vi "Example Toolbar.vi"() -> ()   [LabVIEW 2011, in "Toolbar Control.lvclass"]
doc: "This is an example VI that demonstrates how to use the Toolbar Control object. Run the VI and following the instructions on the front panel.\n\n-------------\nDeveloped by Brian Hoover (hooovahh)"
uses:
  Toolbar Control.lvclass
  Controls/Button State.ctl
  Controls/Horizontal Initialize Settings.ctl
  Controls/Vertical Initialize Settings.ctl
  <userlib>/_OpenG.lib/file/file.llb/Build Path - File Names Array - path__ogtk.vi
  Public Functions/Add Icons From Paths.vi
  Properties/Read Button Pressed Event.vi
  Properties/Read Draw Toolbar Event.vi
  Properties/Write Picture Control Bounds.vi
  Properties/Write Background Color.vi
panel:
  out "Picture":picture
  in  "Top Pane Color":u32(colorbox)
  out "Icon Index":i32
  out "Button State":T1
  out "Button Pressed":string
  in  "Button State":T1
  in  "Button Index":i32
  in  "Set State":bool
  in  "stop":bool
  # "Run this VI.  A toolbar is made using only PNG images for what the button should look like when the mouse is not over the button.\n\nIf there are too many buttons, a More Options button will be on the right to show the rest in a vertical list.  If the vertical list is too large it will show a scrollbar for the remaining buttons.\n\nButtons can be enabled, disabled, or disabled and greyed out.  And the pane color can be changed and buttons will change to match."
  # "Button Pressed Indicators"
  # "Set Button State Controls"
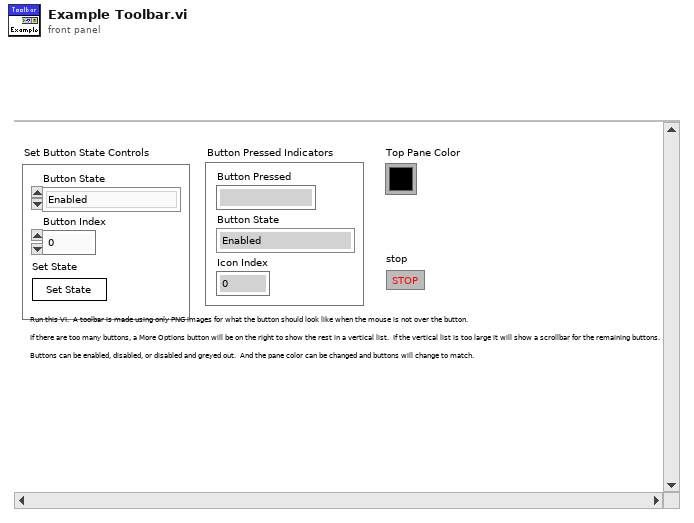
[diagram p1: front panel]
types:
  T1 = typedef "Toolbar Control.lvclass/Button State.ctl" = enum8{"Enabled", "Disabled", "Disabled and Grayed Out"}
  T2 = typedef "Vertical Initialize Settings.ctl" = cluster{"Button Width":i32, "Button Height":i32, "Separator Height":i32}
  T3 = typedef "Horizontal Initialize Settings.ctl" = cluster{"Button Width":i32, "Button Height":i32, "Separator Width":i32, "More Options Width":i32}
  T4 = typedef "LVRectTypeDef.ctl" = cluster{"left":i16, "top":i16, "right":i16, "bottom":i16}
  T5 = typedef "LVPoint32TypeDef.ctl" = cluster{"Horizontal":i32, "Vertical":i32}
  T6 = typedef "Button State.ctl" = enum8{"Enabled", "Disabled", "Disabled and Grayed Out"}
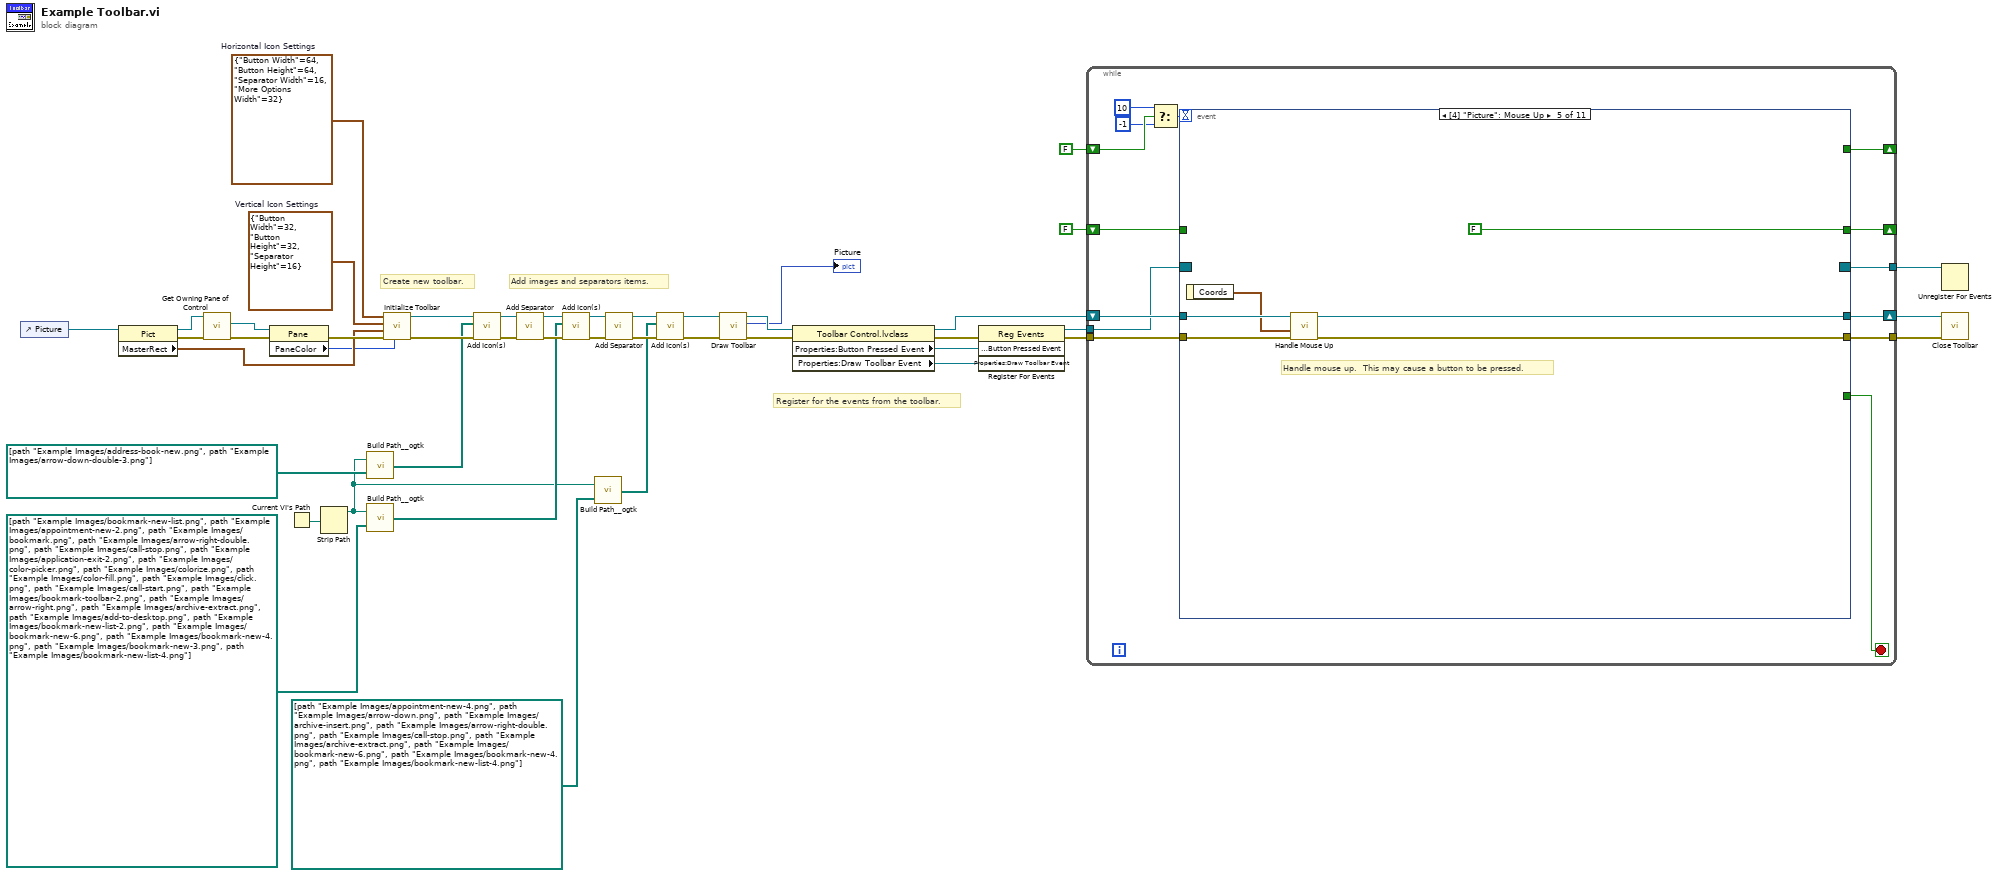
[diagram p0: block diagram]
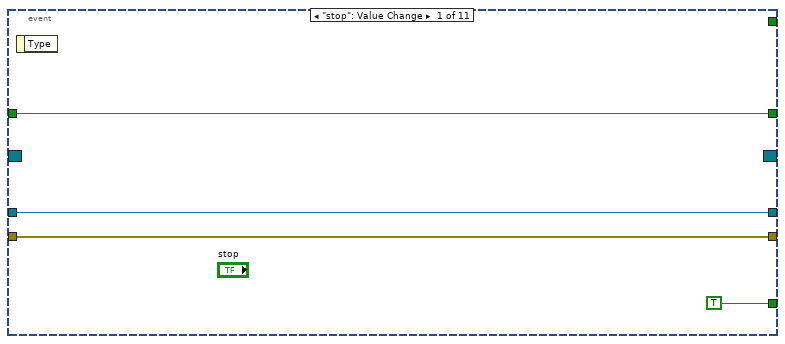
[diagram p2: hidden frame]
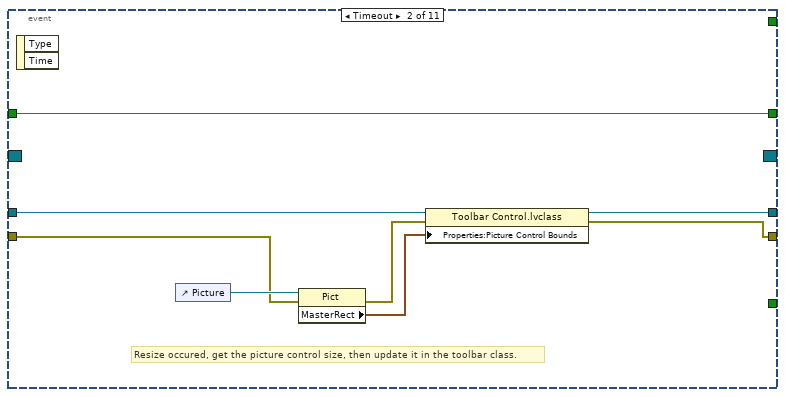
[diagram p3: hidden frame]
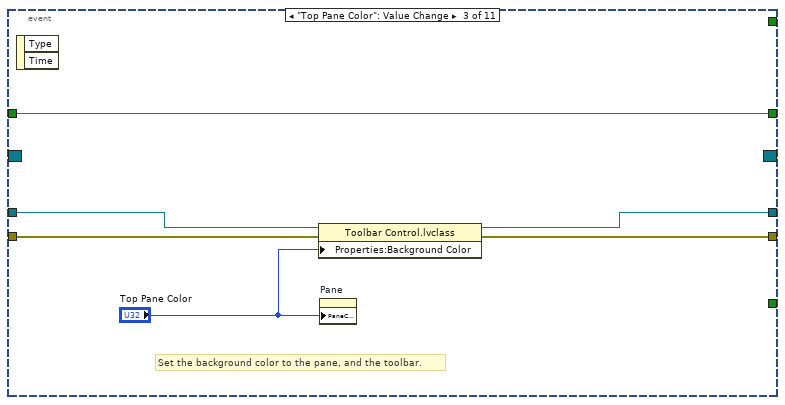
[diagram p4: hidden frame]
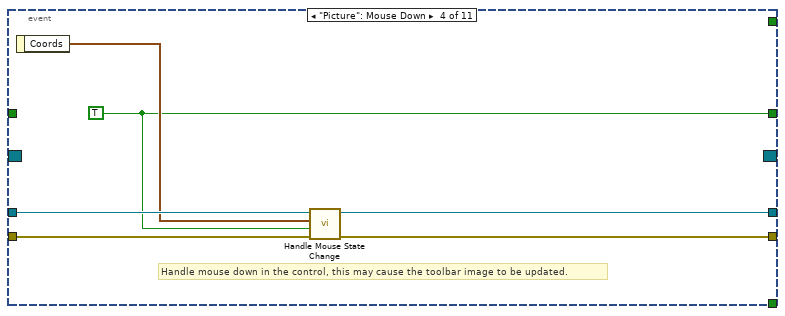
[diagram p5: hidden frame]
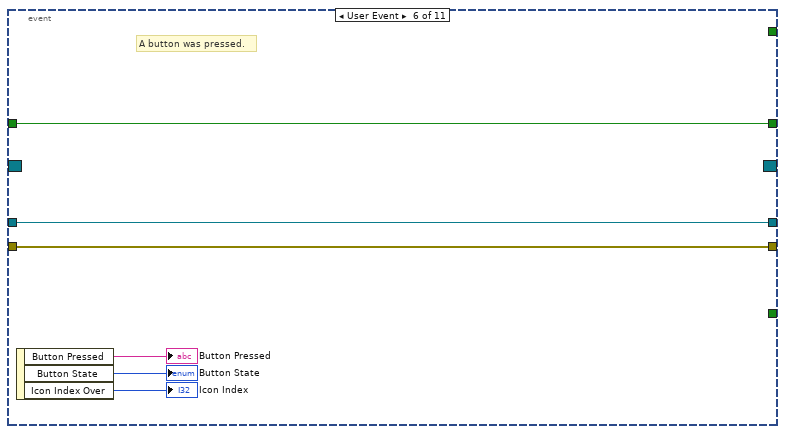
[diagram p6: hidden frame]
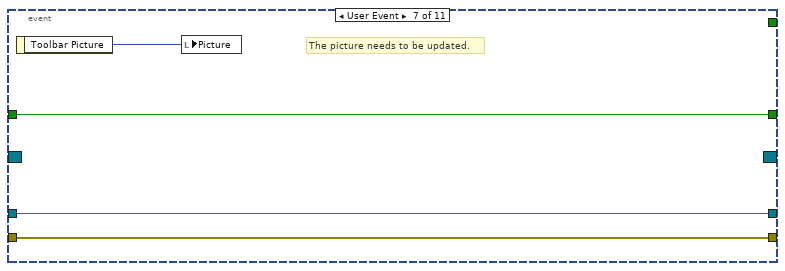
[diagram p7: hidden frame]
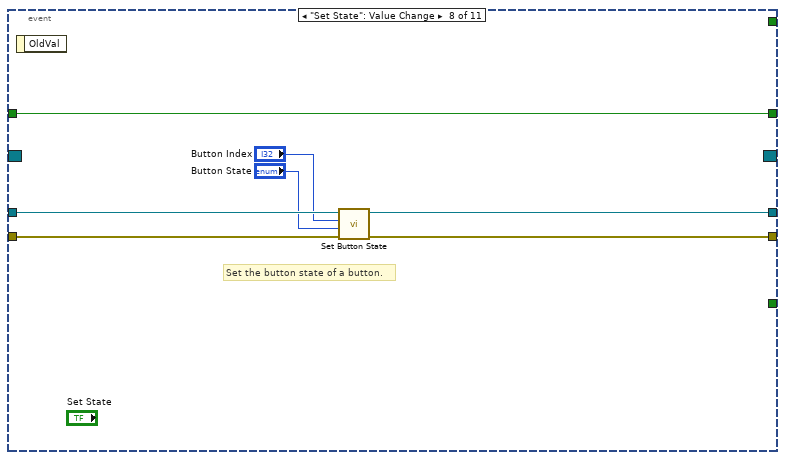
[diagram p8: hidden frame]
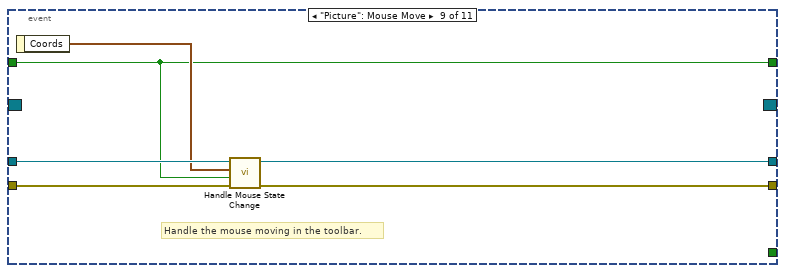
[diagram p9: hidden frame]
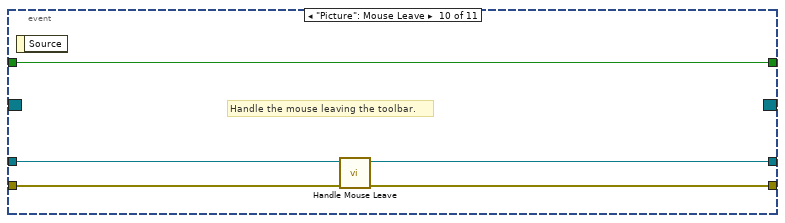
[diagram p10: hidden frame]
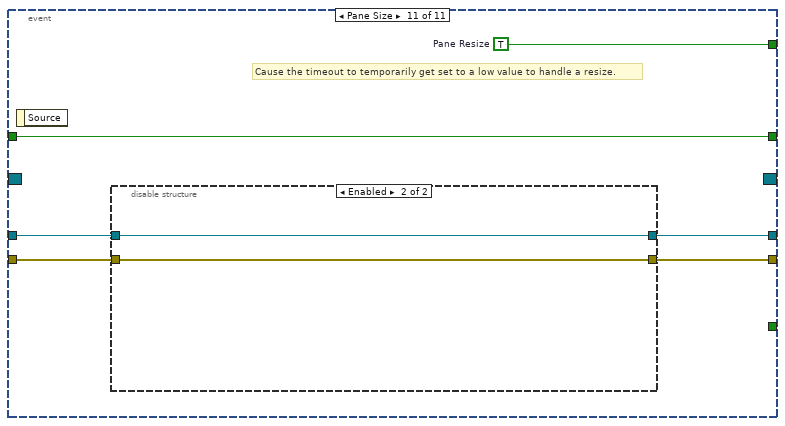
[diagram p11: hidden frame]
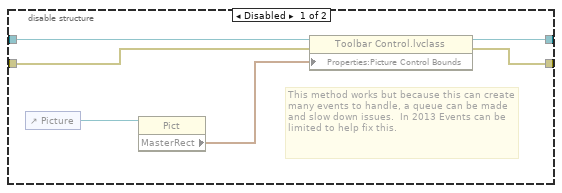
[diagram p12: hidden frame]
diagram:
  w17 = T2 {"Button Width"=32, "Button Height"=32, "Separator Height"=16}  # Vertical Icon Settings
  w18 = T3 {"Button Width"=64, "Button Height"=64, "Separator Width"=16, "More Options Width"=32}  # Horizontal Icon Settings
  # "Register for the events from the toolbar."
  # "Add images and separators items."
  # "Create new toolbar."
  n1 = control-ref of="Picture"() -> (w39:refnum<vi>)
  n2 = property on="Property Node" class="Pict"(reference=w39) -> (reference out=w38:refnum<vi>, error out=w36:errorcluster, "MasterRect"=w33:T4)  [unwired: 1 in]
  n3 = call "Get Owning Pane of Control.vi"("error in (no error)"=w36, "Control Refnum"=w38) -> ("error out"=w35:errorcluster, "Owning Pane"=w37:refnum<vi>)  [unwired: 7 in, 1 out]
  n4 = property class="Pane"(reference=w37, error in=w35) -> (error out=w34:errorcluster, "PaneColor"=w10:u32)  [unwired: 1 out]
  n5 = Current VI's Path() -> (path=w15:path)
  n6 = Strip Path(path=w15) -> (stripped path=w2:path)  [unwired: 1 out]
  n7 = call-poly <userlib>:"Build Path__ogtk.vi"("name or relative path"=path[] [path "Example Images/address-book-new.png", path "Example Images/arrow-down-double-3.png"], "base path"=w2) -> ("appended path"=w11:path[])
  n8 = call-poly <userlib>:"Build Path__ogtk.vi"("name or relative path"=path[] [path "Example Images/bookmark-new-list.png", path "Example Images/appointment-new-2.png", path "Example Images/bookmark.png", path "Example Images/arrow-right-double.png", path "Example Images/call-stop.png", path "Example Images/application-exit-2.png", path "Example Images/color-picker.png", path "Example Images/colorize.png", path "Example Images/color-fill.png", path "Example Images/click.png", path "Example Images/call-start.png", path "Example Images/bookmark-toolbar-2.png", path "Example Images/arrow-right.png", path "Example Images/archive-extract.png", path "Example Images/add-to-desktop.png", path "Example Images/bookmark-new-list-2.png", path "Example Images/bookmark-new-6.png", path "Example Images/bookmark-new-4.png", path "Example Images/bookmark-new-3.png", path "Example Images/bookmark-new-list-4.png"], "base path"=w2) -> ("appended path"=w13:path[])
  n9 = call "Initialize Toolbar.vi"("Background Color"=w10, "error in (no error)"=w34, "Picture Control Bounds"=w33, "Vertical Icon Settings"=w17, "Horizontal Icon Settings"=w18) -> ("error out"=w43:errorcluster, "Toolbar Control out"=w44:refnum<class "Toolbar Control.lvclass">)  [unwired: 5 in]
  n10 = call-poly "Add Icon(s).vi"("error in (no error)"=w43, "Paths"=w11, "Toolbar Control in"=w44) -> ("error out"=w42:errorcluster, "Toolbar Control out"=w31:refnum<class "Toolbar Control.lvclass">)  [unwired: 7 in]
  n11 = call "Add Separator.vi"("error in (no error)"=w42, "Toolbar Control in"=w31) -> ("error out"=w32:errorcluster, "Toolbar Control out"=w30:refnum<class "Toolbar Control.lvclass">)  [unwired: 8 in]
  n12 = call-poly "Add Icon(s).vi"("error in (no error)"=w32, "Paths"=w13, "Toolbar Control in"=w30) -> ("error out"=w8:errorcluster, "Toolbar Control out"=w9:refnum<class "Toolbar Control.lvclass">)  [unwired: 7 in]
  n13 = call-poly <userlib>:"Build Path__ogtk.vi"("name or relative path"=path[] [path "Example Images/appointment-new-4.png", path "Example Images/arrow-down.png", path "Example Images/archive-insert.png", path "Example Images/arrow-right-double.png", path "Example Images/call-stop.png", path "Example Images/archive-extract.png", path "Example Images/bookmark-new-6.png", path "Example Images/bookmark-new-4.png", path "Example Images/bookmark-new-list-4.png"], "base path"=w2) -> ("appended path"=w1:path[])
  n14 = call "Add Separator.vi"("error in (no error)"=w8, "Toolbar Control in"=w9) -> ("error out"=w5:errorcluster, "Toolbar Control out"=w4:refnum<class "Toolbar Control.lvclass">)  [unwired: 8 in]
  n15 = call-poly "Add Icon(s).vi"("error in (no error)"=w5, "Paths"=w1, "Toolbar Control in"=w4) -> ("error out"=w6:errorcluster, "Toolbar Control out"=w7:refnum<class "Toolbar Control.lvclass">)  [unwired: 7 in]
  n16 = call "Draw Toolbar.vi"("error in (no error)"=w6, "Toolbar Control in"=w7) -> ("error out"=w40:errorcluster, "Toolbar Image"=→"Picture":picture, "Toolbar Control out"=w28:refnum<class "Toolbar Control.lvclass">)  [unwired: 7 in]
  n17 = property class="Toolbar Control.lvclass"(reference=w28, error in=w40) -> (reference out=w27:refnum<class "Toolbar Control.lvclass">, error out=w29:errorcluster, "Properties:Button Pressed Event"=w25:refnum<user-event>, "Properties:Draw Toolbar Event"=w24:refnum<user-event>)
  n18 = register-events(error in=w29, w25, w24) -> (reference out=w23:refnum<event-registration>, error out=w26:errorcluster)  [unwired: 1 in]
  n19 = while {
    tunnel: w26 -> [w57]
    shift-right: [w55] -> _
    shift-left: FALSE -> [w56]
    shift-right: [w53] -> w20
    shift-left: w27 -> [w54]
    tunnel: w23 -> [w52]
    tunnel: [w51] -> w21
    tunnel: [w50] -> w19
    shift-right: [w49] -> _
    shift-left: FALSE ("Pane Resize") -> [w48]
    stop <- w58 stop-if-true
    n20 = Select(t=10, s=w48, f=-1) -> (s? t:f=w45:i32)
    n21 = event shown="[4] \"Picture\": Mouse Up" {
      selector: w52 -> [_ _ _ _ _ _ _ _ _ _ _]
      dyn-events: [_ _ _ _ _ _ _ _ _ _ _] -> w51
      timeout: w45 -> [_ _ _ _ _ _ _ _ _ _ _]
      tunnel: [TRUE _ _ _ _ _ _ _ _ _ _] -> w58
      tunnel: w54 -> [w59 w68 w73 w82 w86 w91 w97 w105 w111 w116 w120]
      tunnel: w57 -> [w60 w64 w76 w81 w85 w90 w96 w104 w110 w115 w122]
      tunnel: w56 -> [w61 w65 w75 _ _ w89 w95 w99 w108 w113 w118]
      tunnel: [w61 w65 w75 w79 FALSE w89 w95 w99 w108 w113 w118] -> w55
      tunnel: [w60 w66 w74 w78 w87 w90 w96 w100 w107 w114 w121] -> w50
      tunnel: [w59 w67 w72 w77 w83 w91 w97 w101 w106 w112 w119] -> w53
      tunnel: [_ _ _ _ _ _ _ _ _ _ w117] -> w49
      event "stop": Value Change {
        n22 = event-data() -> ()  [unwired: 1 in, 1 out]
      }
      event Timeout {
        # "Resize occured, get the picture control size, then update it in the toolbar class."
        n23 = event-data() -> ()  [unwired: 1 in, 2 out]
        n24 = control-ref of="Picture"() -> (w70:refnum<vi>)
        n25 = property on="Property Node" class="Pict"(reference=w70, error in=w64) -> (error out=w63:errorcluster, "MasterRect"=w69:T4)  [unwired: 1 out]
        n26 = property class="Toolbar Control.lvclass"(reference=w68, error in=w63, "Properties:Picture Control Bounds"=w69) -> (reference out=w67:refnum<class "Toolbar Control.lvclass">, error out=w66:errorcluster)
      }
      event "Top Pane Color": Value Change {
        # "Set the background color to the pane, and the toolbar."
        n27 = event-data() -> ()  [unwired: 1 in, 2 out]
        n28 = property class="Toolbar Control.lvclass"(reference=w73, error in=w76, "Properties:Background Color"="Top Pane Color") -> (reference out=w72:refnum<class "Toolbar Control.lvclass">, error out=w74:errorcluster)
        n29 = property on="Pane" class="Pane"("PaneColor"="Top Pane Color") -> ()  [unwired: 2 in, 2 out]
      }
      event "Picture": Mouse Down {
        w79 = TRUE
        # "Handle mouse down in the control, this may cause the toolbar image to be updated."
        n30 = event-data() -> ("Coords"=w80:T5)  [unwired: 1 in]
        n31 = call "Handle Mouse State Change.vi"("error in (no error)"=w81, "Mouse Down"=w79, "Mouse Coordinates"=w80, "Toolbar Control in"=w82) -> ("error out"=w78:errorcluster, "Toolbar Control out"=w77:refnum<class "Toolbar Control.lvclass">)  [unwired: 4 in, 2 out]
      }
      event "Picture": Mouse Up {
        # "Handle mouse up.  This may cause a button to be pressed."
        n32 = event-data() -> ("Coords"=w84:T5)  [unwired: 1 in]
        n33 = call "Handle Mouse Up.vi"("error in (no error)"=w85, "Mouse Coordinates"=w84, "Toolbar Control in"=w86) -> ("error out"=w87:errorcluster, "Toolbar Control out"=w83:refnum<class "Toolbar Control.lvclass">)  [unwired: 4 in, 3 out]
      }
      event User Event {
        # "A button was pressed."
        n34 = event-data() -> ("Button Pressed"=→"Button Pressed":string, "Button State"=→"Button State":T6, "Icon Index Over"=→"Icon Index":i32)  [unwired: 1 in]
      }
      event User Event {
        # "The picture needs to be updated."
        n35 = event-data() -> ("Toolbar Picture"=w98:picture)  [unwired: 1 in]
        n36 = local write "Picture"(w98) -> ()
      }
      event "Set State": Value Change {
        # "Set the button state of a button."
        n37 = event-data() -> ()  [unwired: 1 in, 1 out]
        n38 = call "Set Button State.vi"("error in (no error)"=w104, "Button State"="Button State", "Button Index"="Button Index", "Toolbar Control in"=w105) -> ("error out"=w100:errorcluster, "Toolbar Control out"=w101:refnum<class "Toolbar Control.lvclass">)  [unwired: 5 in, 1 out]
      }
      event "Picture": Mouse Move {
        # "Handle the mouse moving in the toolbar."
        n39 = event-data() -> ("Coords"=w109:T5)  [unwired: 1 in]
        n40 = call "Handle Mouse State Change.vi"("error in (no error)"=w110, "Mouse Down"=w108, "Mouse Coordinates"=w109, "Toolbar Control in"=w111) -> ("error out"=w107:errorcluster, "Toolbar Control out"=w106:refnum<class "Toolbar Control.lvclass">)  [unwired: 4 in, 2 out]
      }
      event "Picture": Mouse Leave {
        # "Handle the mouse leaving the toolbar."
        n41 = event-data() -> ()  [unwired: 1 in, 1 out]
        n42 = call "Handle Mouse Leave.vi"("error in (no error)"=w115, "Toolbar Control in"=w116) -> ("error out"=w114:errorcluster, "Toolbar Control out"=w112:refnum<class "Toolbar Control.lvclass">)  [unwired: 7 in, 1 out]
      }
      event Pane Size {
        w117 = TRUE  # Pane Resize
        # "Cause the timeout to temporarily get set to a low value to handle a resize."
        n43 = event-data() -> ()  [unwired: 1 in, 1 out]
        n44 = disable-structure shown="Enabled" {
          disable-tunnel: w122 -> [w128 w129]
          disable-tunnel: [w126 w129] -> w121
          disable-tunnel: w120 -> [w125 w130]
          disable-tunnel: [w124 w130] -> w119
          frame Disabled {
            # "This method works but because this can create many events to handle, a queue can be made and slow down issues.  In 2013 Events can be limited to help fix this."
            n45 = control-ref of="Picture"() -> (w127:refnum<vi>)
            n46 = property on="Property Node" class="Pict"(reference=w127) -> ("MasterRect"=w123:T4)  [unwired: 1 in, 2 out]
            n47 = property class="Toolbar Control.lvclass"(reference=w125, error in=w128, "Properties:Picture Control Bounds"=w123) -> (reference out=w124:refnum<class "Toolbar Control.lvclass">, error out=w126:errorcluster)
          }
          frame Enabled {
          }
        }
      }
    }
  }
  n48 = Unregister For Events(event registration refnum=w21) -> ()  [unwired: 1 in, 1 out]
  n49 = call "Close Toolbar.vi"("error in (no error)"=w19, "Toolbar Control in"=w20) -> ()  [unwired: 9 in, 1 out]
